vi "Read text.vi"(8 "error in (no error)":errorcluster, 11 "TextDecoration in":refnum<class "TextDecoration.lvclass">) -> (0 "error out":errorcluster, 2 "text":string, 3 "TextDecoration out":refnum<class "TextDecoration.lvclass">)   [LabVIEW 2023, in "TLC_Scripto.lvlib" / "TextDecoration.lvclass"]
uses:
  TextDecoration.lvclass
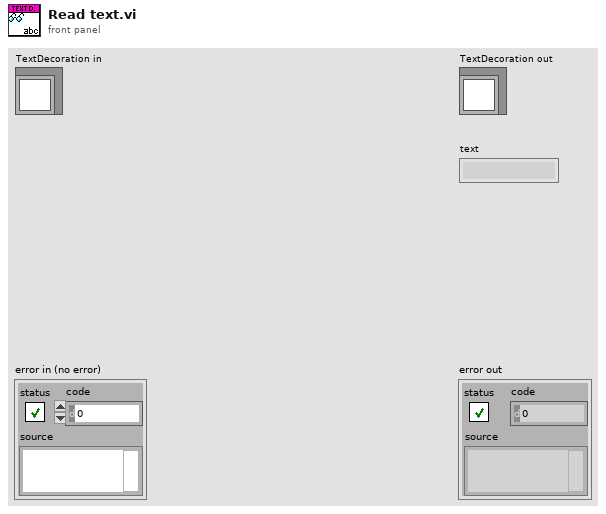
[diagram p1: front panel]
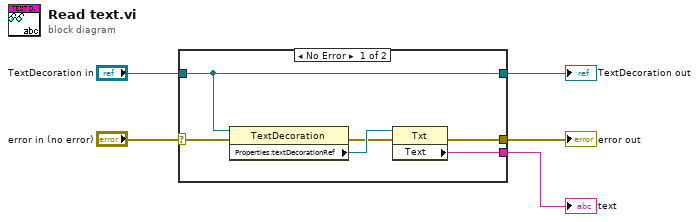
[diagram p0: block diagram]
diagram:
  n1 = case shown="No Error" "error in (no error)" {
    selector: "error in (no error)" -> [w7 w12]
    tunnel: [w6 w12] -> w4
    tunnel: [w9 w13] -> w2
    tunnel: "TextDecoration in" -> [w9 w13]
    tunnel: [w8 _] -> w1
    frame No Error {
      n2 = property class="TextDecoration"(reference=w9, error in=w7) -> (error out=w10:errorcluster, "Properties:textDecorationRef"=w11:refnum<vi>)  [unwired: 1 out]
      n3 = property class="Txt"(reference=w11, error in=w10) -> (error out=w6:errorcluster, "Text"=w8:string)  [unwired: 1 out]
    }
    frame Error {
    }
  }
  "error out" <- w4
  "TextDecoration out" <- w2
  "text" <- w1
